vi "T to Delta.vi"(5 "H":dbl=20.0 format="%#_6pT", 7 "Hc2 at T":dbl=20.0 format="%#_6pT", 9 "Delta Tc factor":dbl=1.764, 10 "Tc":dbl=20.0 format="%#_6pK", 11 "T":dbl) -> (1 "BSC Delta T H":dbl=0.003040195174884819 format="%#_6peV", 2 "BSC Delta T":dbl=0.003040195174884819 format="%#_6peV", 3 "BSC Delta 0":dbl=0.003040195174884819 format="%#_6peV")   [LabVIEW 2021]
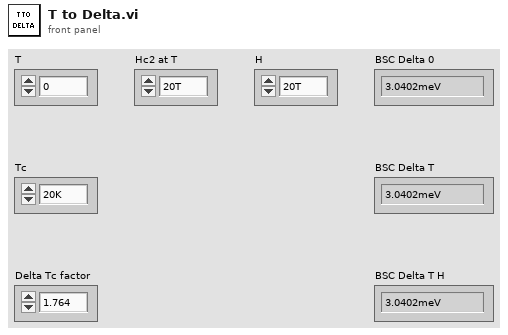
[diagram p1: front panel]
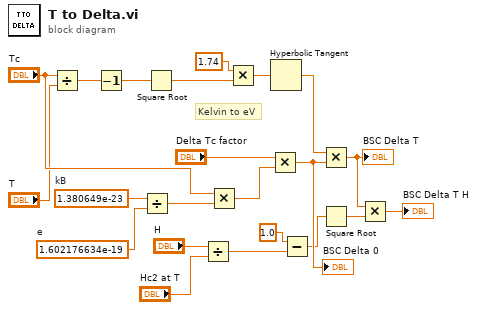
[diagram p0: block diagram]
diagram:
  w19 = 1.602176634e-19  # e
  w20 = 1.380649e-23  # kB
  # "Kelvin to eV"
  n1 = Divide(x="Tc", y="T") -> (x/y=w15:dbl)
  n2 = Decrement(x=w15) -> (x-1=w14:dbl)
  n3 = Divide(x=w20, y=w19) -> (x/y=w21:dbl)
  n4 = Square Root(x=w14) -> (sqrt(x)=w13:dbl)
  n5 = Divide(x="H", y="Hc2 at T") -> (x/y=w6:dbl)
  n6 = Multiply(x="Tc", y=w21) -> (x*y=w22:dbl)
  n7 = Multiply(x=1.74, y=w13) -> (x*y=w11:dbl)
  n8 = Multiply(x="Delta Tc factor", y=w22) -> (x*y=w10:dbl)
  "BSC Delta 0" <- w10
  n9 = Hyperbolic Tangent(1:w11) -> (0:w9:dbl)
  n10 = Subtract(x=1.0, y=w6) -> (x-y=w4:dbl)
  n11 = Multiply(x=w9, y=w10) -> (x*y=w2:dbl)
  "BSC Delta T" <- w2
  n12 = Square Root(x=w4) -> (sqrt(x)=w3:dbl)
  n13 = Multiply(x=w2, y=w3) -> (x*y=→"BSC Delta T H":dbl)
